vi "Measurement Example.vi"(8 "error in (no error)":errorcluster, 11 "UDP in":refnum<class "UDP.lvclass">) -> (0 "error out":errorcluster, 3 "UDP out":refnum<class "UDP.lvclass">)   [LabVIEW 2020, in "Plugin Instrument Driver.lvlib" / "UDP.lvclass"]
doc: "Initialize connection, Read Measurement & Close the connection"
uses:
  UDP.lvclass
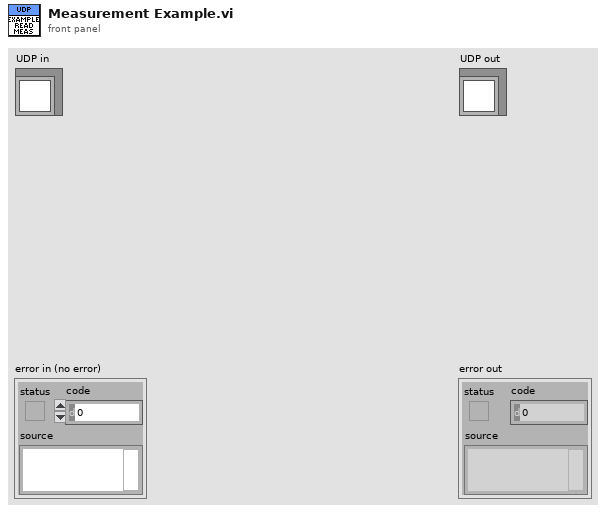
[diagram p1: front panel]
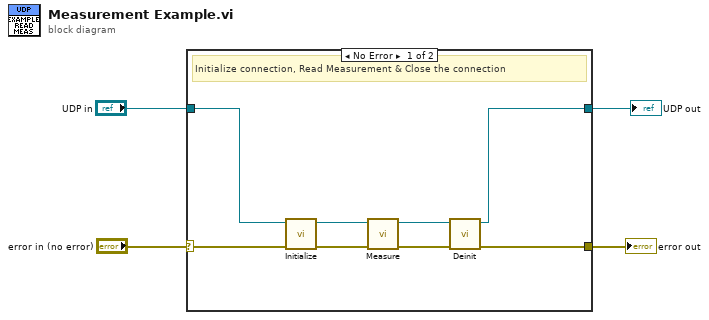
[diagram p0: block diagram]
diagram:
  n1 = case shown="No Error" "error in (no error)" {
    selector: "error in (no error)" -> [w8 w14]
    tunnel: [w7 w14] -> w3
    tunnel: [w5 w13] -> w1
    tunnel: "UDP in" -> [w6 w13]
    frame No Error {
      # "Initialize connection, Read Measurement & Close the connection"
      n2 = call-dynamic "Initialize.vi"("error in"=w8, "UDP in"=w6) -> ("error out"=w11:errorcluster, "UDP out"=w12:refnum<class "UDP.lvclass">)  [unwired: 8 in]
      n3 = call-dynamic "Measure.vi"("error in"=w11, "UDP in"=w12) -> ("error out"=w9:errorcluster, "UDP out"=w10:refnum<class "UDP.lvclass">)  [unwired: 7 in, 1 out]
      n4 = call-dynamic "Deinit.vi"("error in"=w9, "UDP in"=w10) -> ("error out"=w7:errorcluster, "UDP out"=w5:refnum<class "UDP.lvclass">)  [unwired: 8 in]
    }
    frame Error {
    }
  }
  "error out" <- w3
  "UDP out" <- w1
